vi "CtrlTrain_Analog_HighLowLimit.vi"(9 "Lo_Limit":dbl=-100.0, 10 "Hi_Limit":dbl=100.0, 11 "Input":dbl) -> (3 "Output":dbl)   [LabVIEW 2019, in "CtrlTrainingLibary_Protected.lvlib"]
doc: "This VI rate limits the input. This VI remembers the last output. If there are multiple VI that set the same output, use the RateLimit2 VI. This one has an input connection to send the last output value."
uses:
  CtrlTrainingLibary_Protected.lvlib
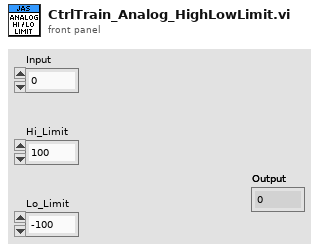
[diagram p1: front panel]
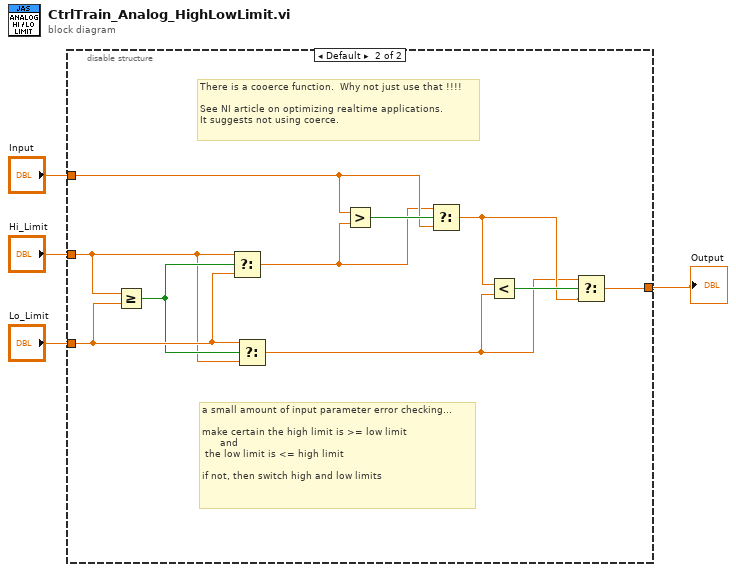
[diagram p0: block diagram]
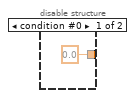
[diagram p2: hidden frame]
diagram:
  n1 = disable-structure shown="Default" {
    disable-tunnel: "Input" -> [_ w13]
    disable-tunnel: [0.0 ("Input") w11] -> w3
    disable-tunnel: "Lo_Limit" -> [_ w8]
    disable-tunnel: "Hi_Limit" -> [_ w6]
    frame condition #0 {
    }
    frame condition #1 (active) {
      # "There is a cooerce function.  Why not just use that !!!!\n\nSee NI article on optimizing realtime applications.\nIt suggests not using coerce."
      # "a small amount of input parameter error checking...\n\nmake certain the high limit is >= low limit\n      and\n the low limit is <= high limit\n\nif not, then switch high and low limits"
      n2 = Greater Or Equal?(x=w6, y=w8) -> (x >= y?=w7:bool)
      n3 = Select(t=w6, s=w7, f=w8) -> (s? t:f=w10:dbl)
      n4 = Select(t=w8, s=w7, f=w6) -> (s? t:f=w9:dbl)
      n5 = Greater?(x=w13, y=w10) -> (0:w15:bool)
      n6 = Select(t=w10, s=w15, f=w13) -> (s? t:f=w12:dbl)
      n7 = Less?(x=w12, y=w9) -> (x < y?=w14:bool)
      n8 = Select(t=w9, s=w14, f=w12) -> (s? t:f=w11:dbl)
    }
  }
  "Output" <- w3
